vi "Status example.vi"(8 "error in (no error)":errorcluster) -> (0 "error out":errorcluster)   [LabVIEW 2017]
uses:
  <vilib>/LVH/i3 JSON/JSON Parsing/Get Object Parameter Files/Get Object Parameter - Numeric.vi
  <vilib>/LVH/i3 JSON/JSON Parsing/Get Object Parameter Files/Get Object Parameter - String.vi
  <vilib>/LVH/i3 JSON/JSON Parsing/Get Object Parameter Files/Get Object Parameter - Object.vi
  <vilib>/LVH/i3 JSON/i3-json.lvlib
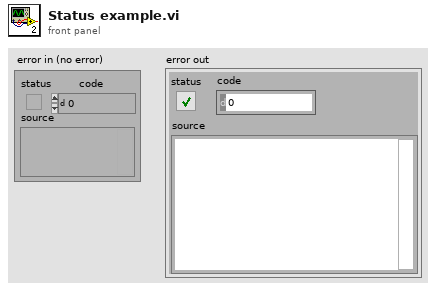
[diagram p1: front panel]
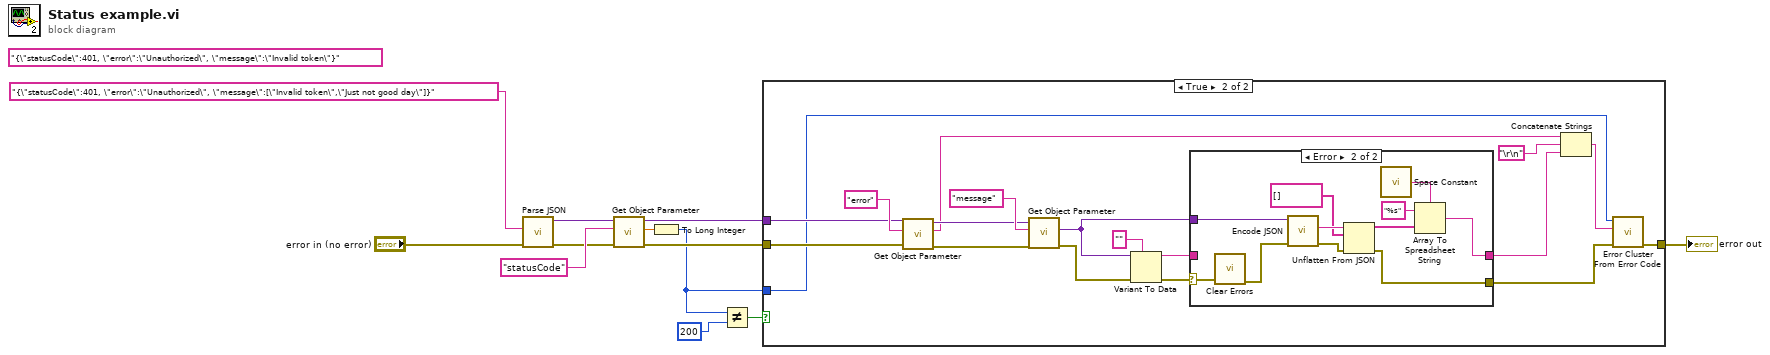
[diagram p0: block diagram]
diagram:
  (unwired) "{\"statusCode\":401, \"error\":\"Unauthorized\", \"message\":\"Invalid token\"}"
  n1 = call <vilib>:"Parse JSON.vi"("error in (no error)"="error in (no error)", "JSON String"="{\"statusCode\":401, \"error\":\"Unauthorized\", \"message\":[\"Invalid token\",\"Just not good day\"]}") -> ("error out"=w6:errorcluster, "JSON Tree"=w8:variant)  [unwired: 6 in, 2 out]
  n2 = call-poly <vilib>:"Get Object Parameter.vi"("error in (no error)"=w6, "Parameter Name"="statusCode", "JSON Tree In (JSON Object)"=w8) -> ("error out"=w5:errorcluster, "Double Value"=w11:dbl, "JSON Tree Out Passthrough"=w4:variant)  [unwired: 5 in, 1 out]
  n3 = To Long Integer(number=w11) -> (32bit integer=w3:i32)
  n4 = Not Equal?(x=w3, y=200) -> (x != y?=w9:bool)
  n5 = case shown="True" w9 {
    tunnel: w4 -> [_ w25]
    tunnel: w5 -> [w13 w24]
    tunnel: w3 -> [_ w22]
    tunnel: [w13 w31] -> w2
    frame False {
    }
    frame True {
      n6 = call-poly <vilib>:"Get Object Parameter.vi"("error in (no error)"=w24, "Parameter Name"="error", "JSON Tree In (JSON Object)"=w25) -> ("error out"=w27:errorcluster, "String Value"=w26:string, "JSON Tree Out Passthrough"=w28:variant)  [unwired: 5 in, 1 out]
      n7 = call-poly <vilib>:"Get Object Parameter.vi"("error in (no error)"=w27, "Parameter Name"="message", "JSON Tree In (JSON Object)"=w28) -> ("error out"=w19:errorcluster, "JSON Object"=w16:variant)  [unwired: 5 in, 2 out]
      n8 = Variant To Data(error in=w19, type="", Variant=w16) -> (data=w17:string, error out=w18:errorcluster)
      n9 = case shown="Error" w18 {
        selector: w18 -> [w32 w37]
        tunnel: w17 -> [w33 _]
        tunnel: [w33 w34] -> w15
        tunnel: w16 -> [_ w38]
        tunnel: [w32 w35] -> w14
        frame No Error {
        }
        frame Error {
          n10 = call <vilib>:"Clear Errors.vi"("error in (no error)"=w37) -> ("error out"=w36:errorcluster)  [unwired: 5 in, 1 out]
          n11 = call <vilib>:"Encode JSON.vi"("error in (no error)"=w36, "JSON Tree"=w38) -> ("error out"=w42:errorcluster, "String"=w41:string)  [unwired: 4 in]
          n12 = Unflatten From JSON(JSON string=w41, type and defaults=string[] [], error in (no error)=w42) -> (value=w43:string[], error out=w35:errorcluster)  [unwired: 4 in]
          n13 = call <vilib>:"Space Constant.vi"() -> ("String"=w44:string)
          n14 = Array To Spreadsheet String(delimiter (Tab)=w44, array=w43, 3:"%s" ("format string")) -> (spreadsheet string=w34:string)
        }
      }
      n15 = Concatenate Strings(w26, "\r\n", w15) -> (w23:string)
      n16 = call <vilib>:"Error Cluster From Error Code.vi"("error in (no error)"=w14, "error message (\"\")"=w23, "error code (0)"=w22) -> ("error out"=w31:errorcluster)  [unwired: 6 in]
    }
  }
  "error out" <- w2
